vi "Intensity_png.vi"(3 "No of Contours":i32=20, 4 "Job Directory":path=path "/Lacie_20/paulhayden/Documents/EnFlo bits/EnFlo Tun Vel profiles/View_LDA data.tpt", 5 "Intensity Graph":dbl[][](graph)) -> ()   [LabVIEW 2018]
uses:
  Results_plotter_Global.vi
panel:
  out "Folders":string[](array[string])
  out "String":string
  in  "Added labels":i32[](listbox)
  in  "Z Min":dbl=0.97
  in  "Z Max":dbl=1.07
  in  "Save Automatically?":bool
  in  "Auto scale Intensity":bool=TRUE
  in  "Colour":bool=TRUE
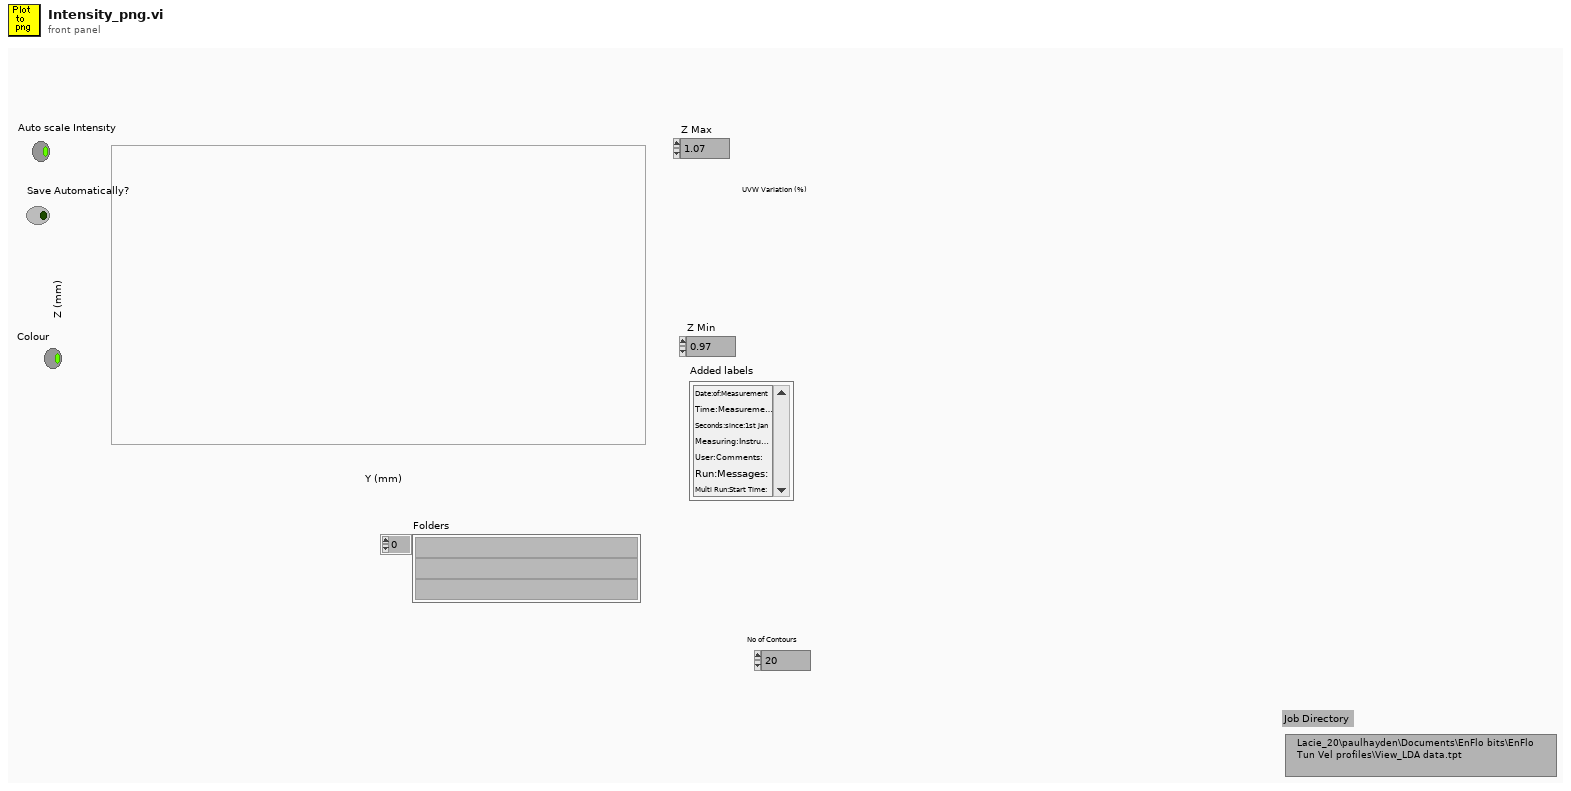
[diagram p1: front panel]
types:
  T1 = typedef "imagedata.ctl" = cluster{"image type":i32, "image depth":i32, "image":u8[], "mask":u8[], "colors":u32[], "Rectangle":cluster{"left":i16, "top":i16, "right":i16, "bottom":i16}}
  T2 = cluster{"left":i16, "top":i16, "right":i16, "bottom":i16}
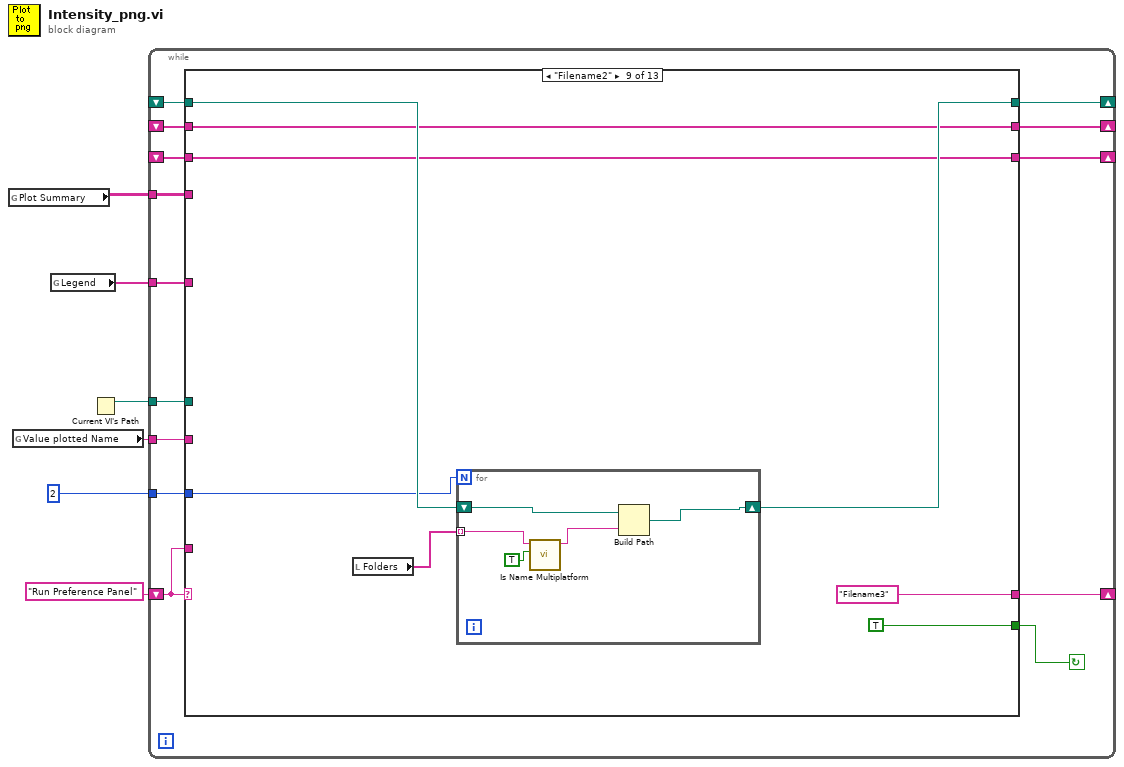
[diagram p0: block diagram]
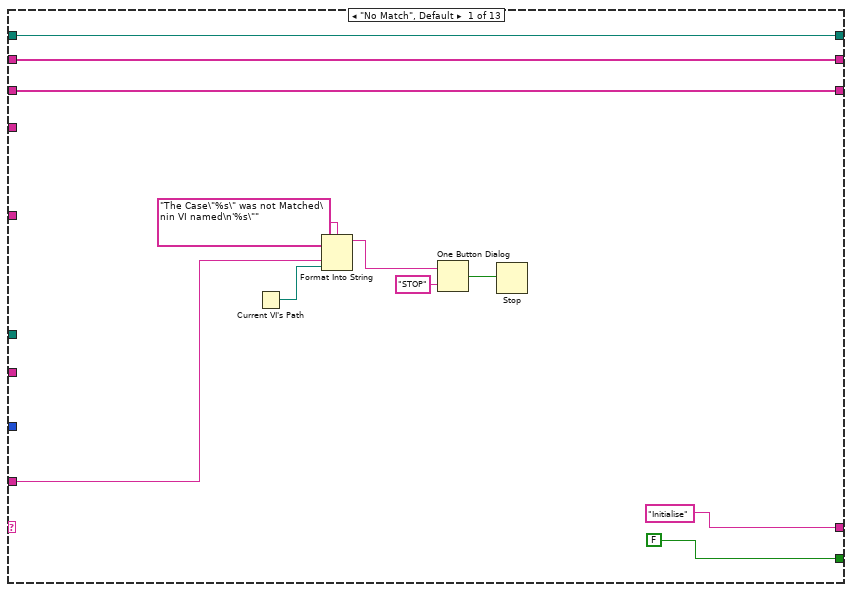
[diagram p2: hidden frame]
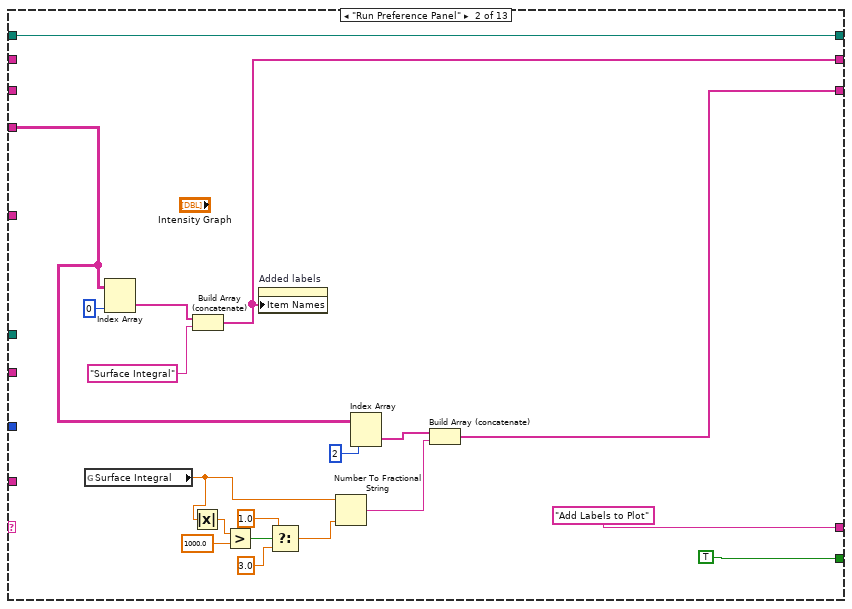
[diagram p3: hidden frame]
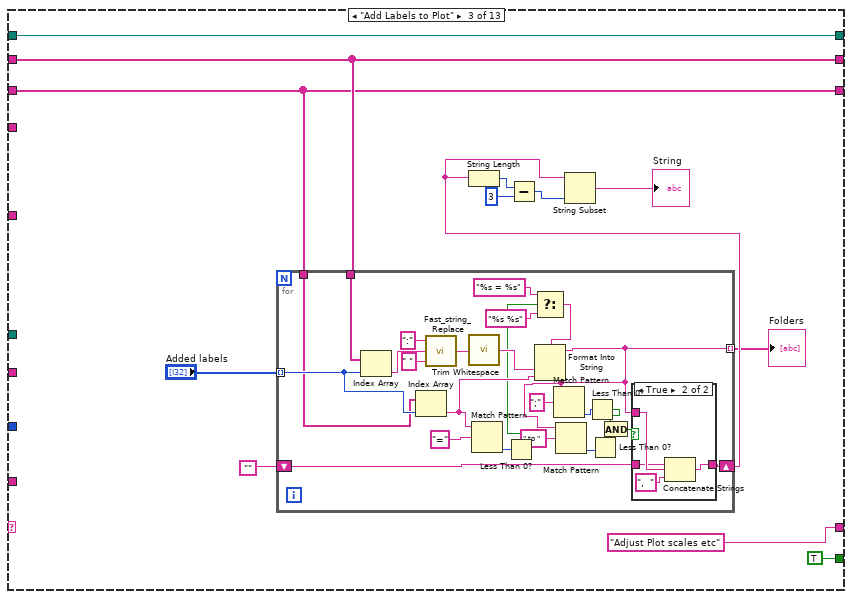
[diagram p4: hidden frame]
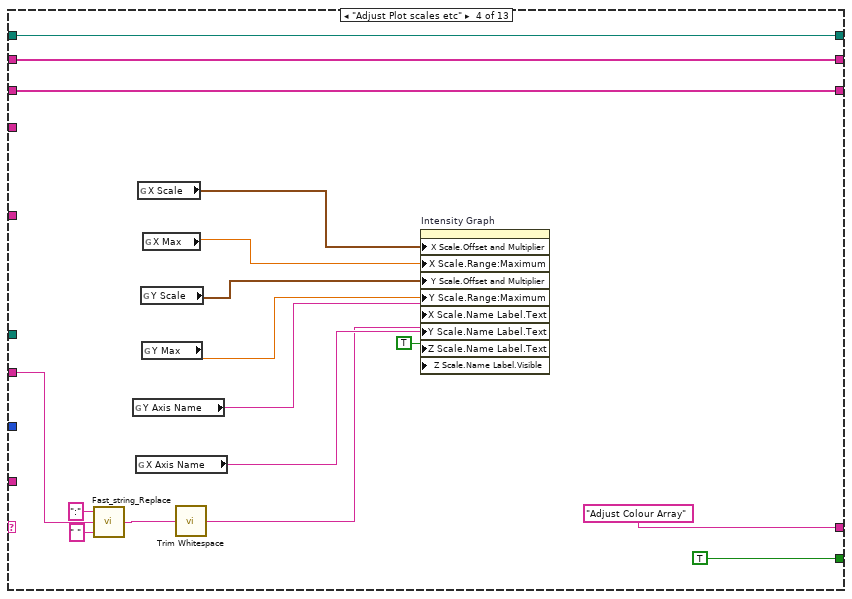
[diagram p6: hidden frame]
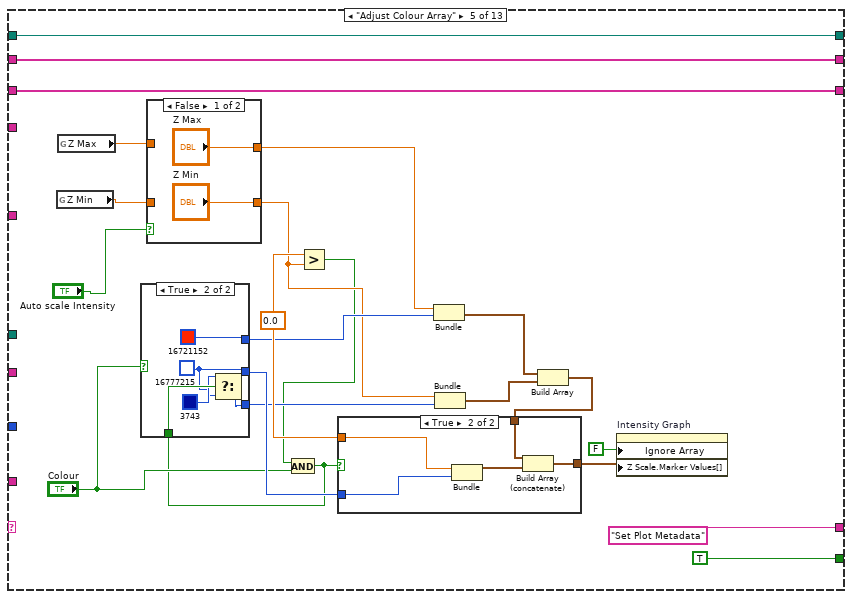
[diagram p7: hidden frame]
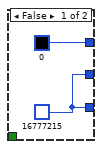
[diagram p8: hidden frame]
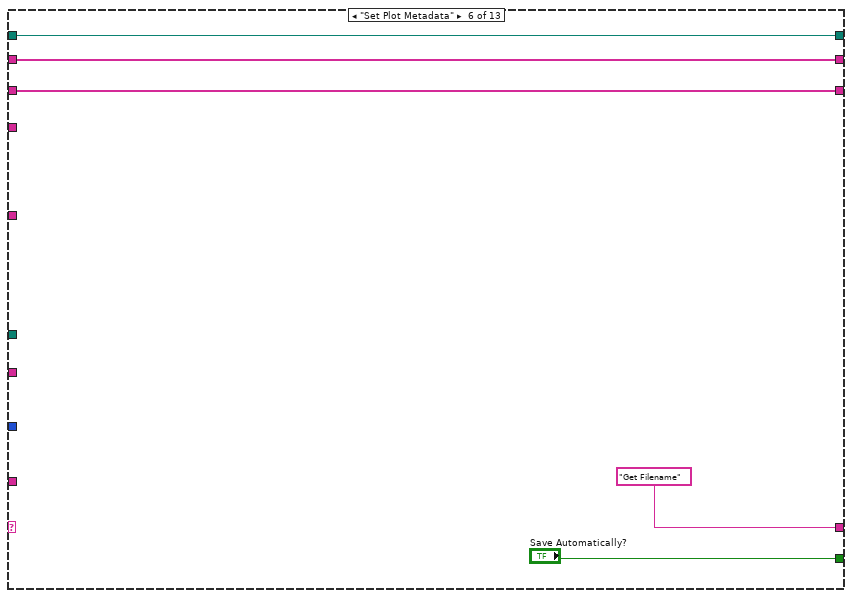
[diagram p11: hidden frame]
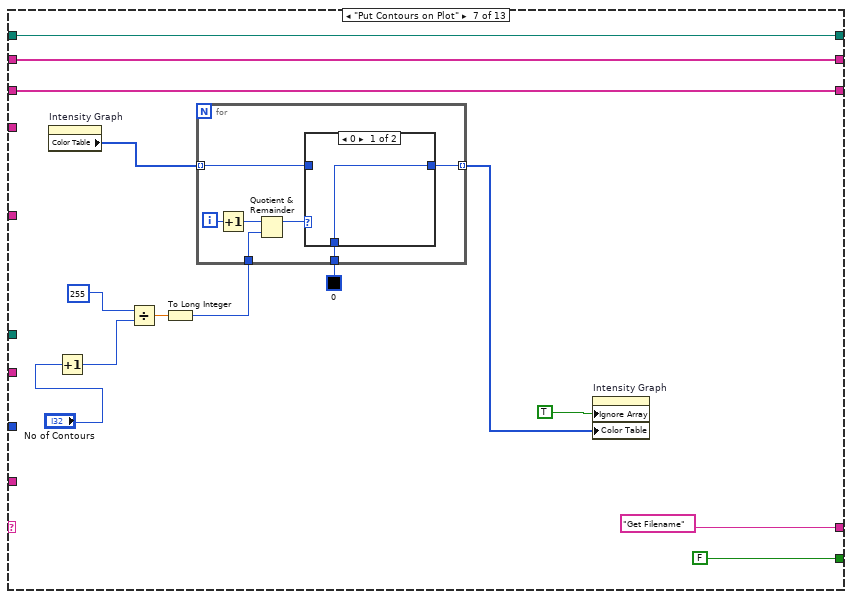
[diagram p12: hidden frame]
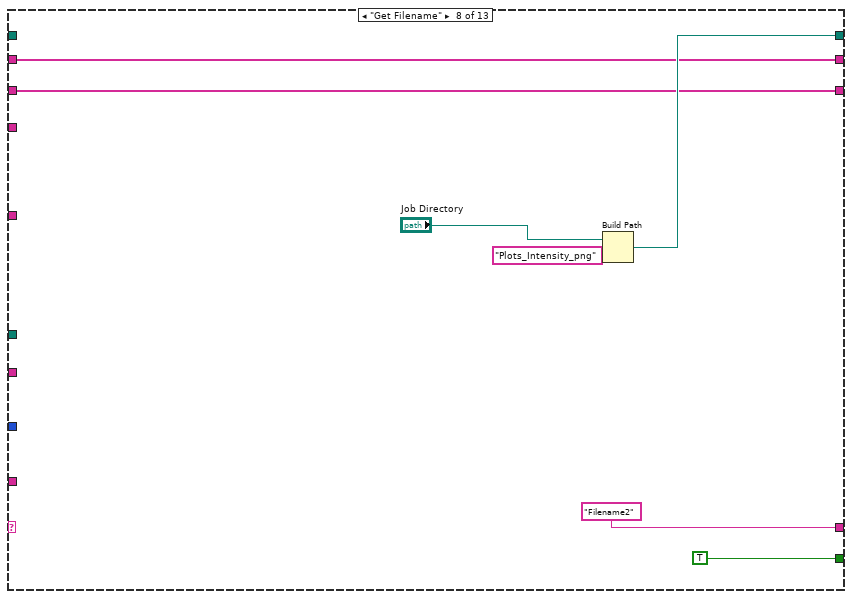
[diagram p14: hidden frame]
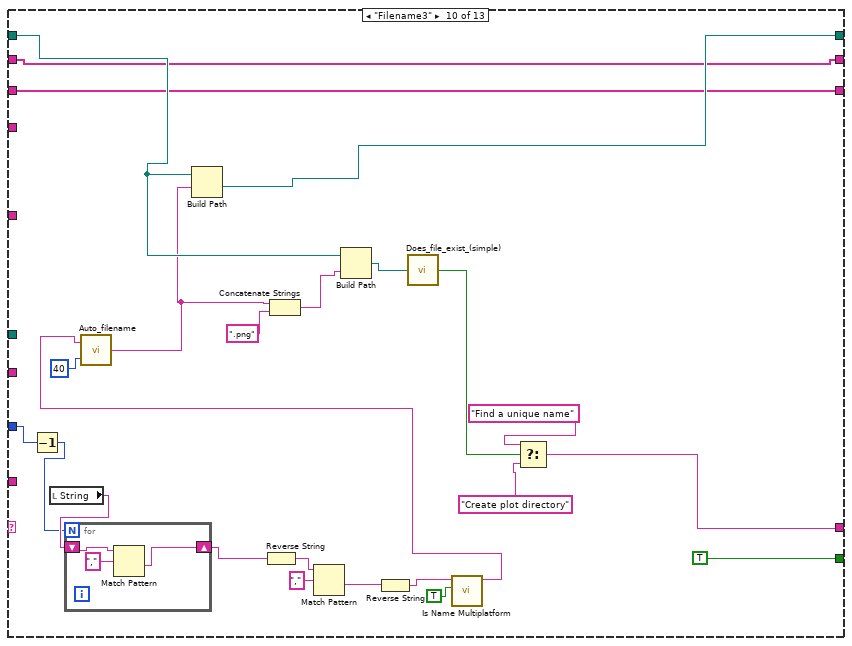
[diagram p15: hidden frame]
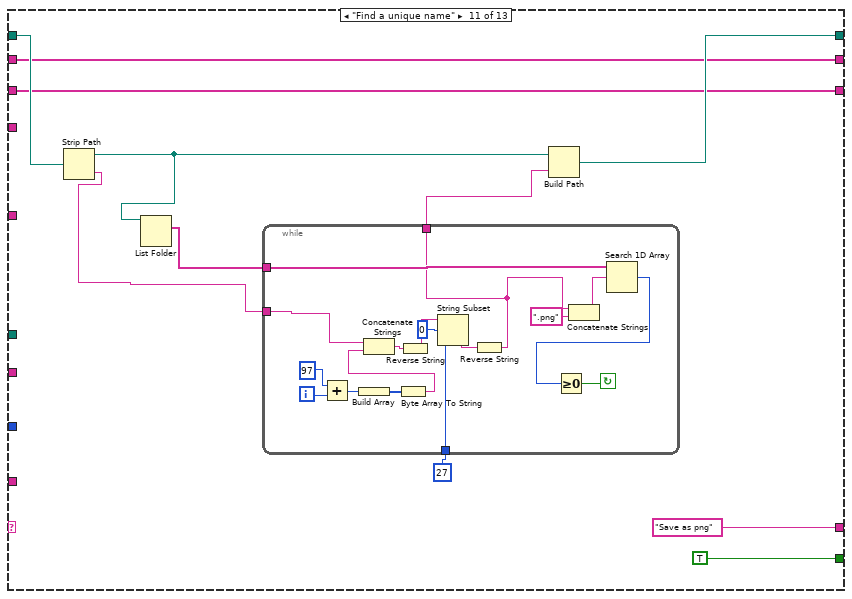
[diagram p16: hidden frame]
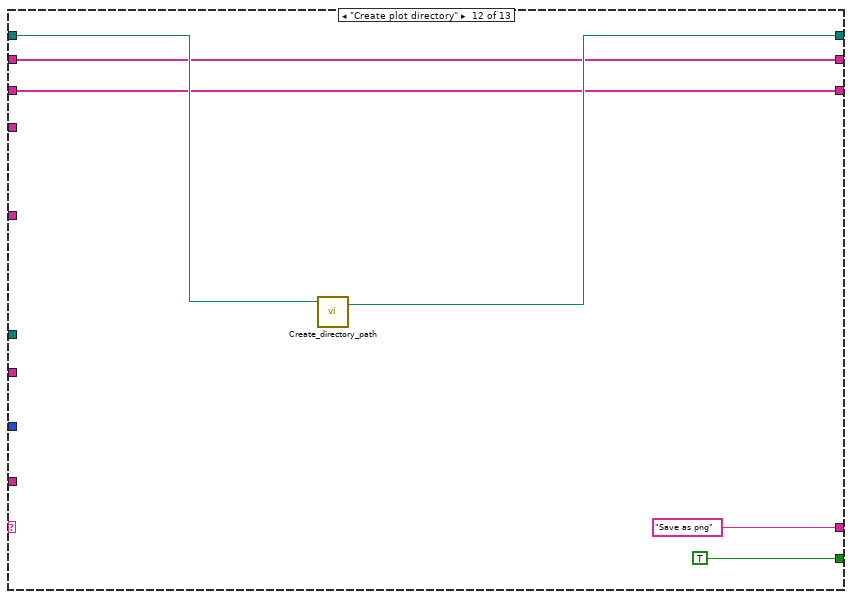
[diagram p17: hidden frame]
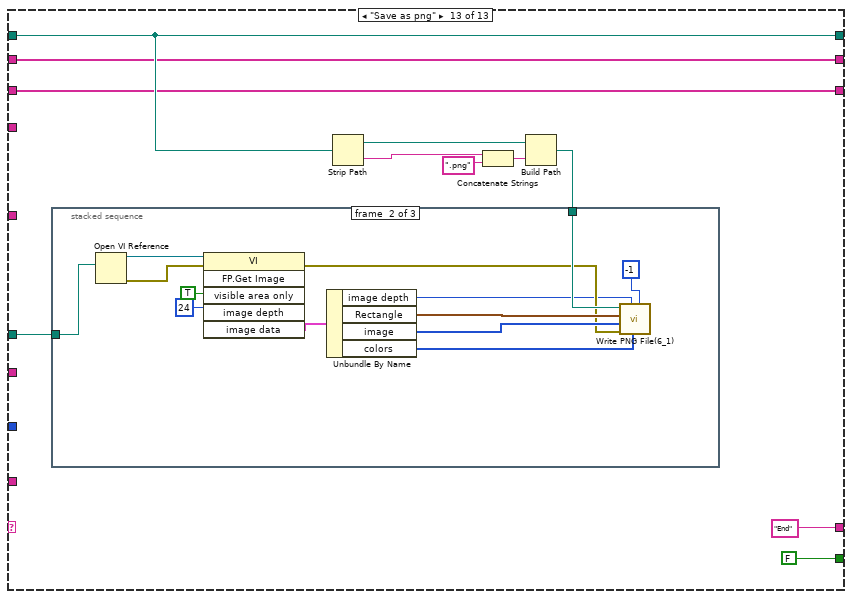
[diagram p18: hidden frame]
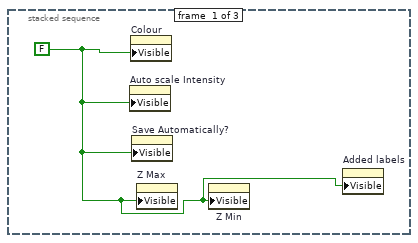
[diagram p19: hidden frame]
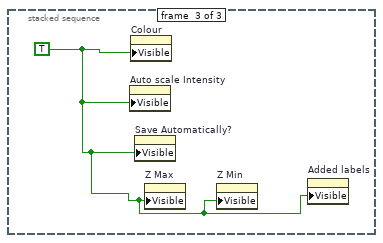
[diagram p20: hidden frame]
diagram:
  n1 = global read "Results_plotter_Global.vi" "Plot Summary"() -> (w2:string[][])
  n2 = global read "Results_plotter_Global.vi" "Value plotted Name"() -> (w4:string)
  n3 = global read "Results_plotter_Global.vi" "Legend"() -> (w3:string[])
  n4 = Current VI's Path() -> (path=w5:path)
  n5 = while {
    shift-left: "Run Preference Panel" -> [w18]
    shift-right: [w19] -> _
    tunnel: w5 -> [w17]
    shift-right: [w16] -> _
    shift-left: _ -> [w15]
    tunnel: w4 -> [w14]
    tunnel: w3 -> [w13]
    tunnel: w2 -> [w12]
    tunnel: 2 -> [w11]
    shift-right: [w10] -> _
    shift-left: _ -> [w8]
    shift-right: [w9] -> _
    shift-left: _ -> [w7]
    stop <- w20 continue-if-true
    n6 = case shown="\"Filename2\"" w18 {
      tunnel: [FALSE TRUE TRUE ("Top Level") TRUE ("Top Level") TRUE ("Top Level") "Save Automatically?" FALSE ("Top Level") TRUE ("Top Level") TRUE ("Top Level") TRUE ("Top Level") TRUE ("Top Level") TRUE ("Top Level") FALSE ("Top Level")] -> w20
      tunnel: ["Initialise" "Add Labels to Plot" "Adjust Plot scales etc" "Adjust Colour Array" "Set Plot Metadata" "Get Filename" "Get Filename" "Filename2" "Filename3" w218 "Save as png" "Save as png" "End"] -> w19
      tunnel: w18 -> [w26 _ _ _ _ _ _ _ _ _ _ _ _]
      tunnel: w17 -> [_ _ _ _ _ _ _ _ _ _ _ _ w268]
      tunnel: [w23 w48 w62 w101 w121 w153 w157 w182 w188 w219 w229 w255 w266] -> w16
      tunnel: w15 -> [w23 w48 w62 w101 w121 w153 w157 _ w190 w220 w230 w256 w266]
      tunnel: w14 -> [_ _ _ w100 _ _ _ _ _ _ _ _ _]
      tunnel: w13 -> [_ _ _ _ _ _ _ _ _ _ _ _ _]
      tunnel: w12 -> [_ w42 _ _ _ _ _ _ _ _ _ _ _]
      tunnel: w11 -> [_ _ _ _ _ _ _ _ w187 w204 _ _ _]
      tunnel: [w22 w44 w52 w95 w112 w151 w156 w179 w186 w202 w226 w254 w262] -> w10
      tunnel: [w21 w39 w51 w94 w111 w150 w155 w178 w185 w201 w225 w253 w261] -> w9
      tunnel: w8 -> [w22 _ w52 w95 w112 w151 w156 w179 w186 w202 w226 w254 w262]
      tunnel: w7 -> [w21 _ w51 w94 w111 w150 w155 w178 w185 w201 w225 w253 w261]
      frame "No Match", Default {
        n7 = Current VI's Path() -> (path=w25:path)
        n8 = Format Into String(format string="The Case\"%s\" was not Matched\nin VI named\n'%s\"" ("Format String"), w26, w25) -> (resulting string=w29:string)  [unwired: 2 in, 1 out]
        n9 = One Button Dialog(message=w29, button name ("OK")="STOP") -> (true=w27:bool)
        n10 = Stop(stop? (T)=w27) -> ()
      }
      frame "Run Preference Panel" {
        n11 = global read "Results_plotter_Global.vi" "Surface Integral"() -> (w33:dbl)
        n12 = Index Array(array=w42, index (col)=0 ("disabled index (col)")) -> (element=w46:string[])  [unwired: 1 in]
        n13 = Absolute Value(x=w33) -> (abs(x)=w32:dbl)
        n14 = Build Array (concatenate)(w46, "Surface Integral" ("Output String")) -> (w44:string[])
        n15 = Greater?(x=w32, y=1000.0) -> (0:w37:bool)
        n16 = property on="Added labels" class="LstBox (strict)"("Item Names"=w44) -> ()  [unwired: 2 in, 2 out]
        n17 = Select(t=1.0, s=w37, f=3.0) -> (s? t:f=w36:dbl)
        n18 = Number To Fractional String(number=w33, precision (6)=w36) -> (F-format string=w41:string)  [unwired: 2 in]
        n19 = Index Array(array=w42, index (col)=2 ("disabled index (col)")) -> (element=w40:string[])  [unwired: 1 in]
        n20 = Build Array (concatenate)(w40, w41) -> (w39:string[])
      }
      frame "Add Labels to Plot" {
        n21 = for {
          tunnel: "Added labels" -> [w87] mode=indexing
          tunnel: w52 -> [w88]
          shift-right: [w79] -> w55
          shift-left: "" -> [w80]
          tunnel: [w65] -> w53 mode=indexing
          tunnel: w51 -> [w64]
          n22 = Index Array(array=w88, index=w87) -> (element=w84:string)
          n23 = Index Array(array=w64, index=w87) -> (element=w78:string)
          n24 = call "Fast_string_Replace.vi"("Replace match with:"=" ", "Input String"=w84, "regular expression"=":") -> ("Output String"=w83:string)  [unwired: 2 out]
          n25 = call <vilib>:"Trim Whitespace.vi"("string"=w83) -> ("trimmed string"=w82:string)  [unwired: 1 in]
          n26 = Match Pattern(string=w78, regular expression="=") -> (offset past match=w76:i32)  [unwired: 4 out]
          n27 = Less Than 0?(x=w76) -> (x < 0?=w75:bool)
          n28 = Select(t="%s = %s" ("format string"), s=w75, f="%s %s" ("format string")) -> (s? t:f=w72:string)
          n29 = Format Into String(format string=w72, w82, w78) -> (resulting string=w65:string)  [unwired: 2 in, 1 out]
          n30 = Match Pattern(string=w65, regular expression=";") -> (offset past match=w70:i32)  [unwired: 4 out]
          n31 = Match Pattern(string=w65, regular expression=" to ") -> (offset past match=w69:i32)  [unwired: 4 out]
          n32 = Less Than 0?(x=w70) -> (x < 0?=w67:bool)
          n33 = Less Than 0?(x=w69) -> (x < 0?=w68:bool)
          n34 = And(x=w67, y=w68) -> (x .and. y?=w66:bool)
          n35 = case shown="True" w66 {
            tunnel: w80 -> [w89 w91]
            tunnel: [w89 w92] -> w79
            tunnel: w65 -> [_ w93]
            frame False {
            }
            frame True {
              n36 = Concatenate Strings(w91, w93, ",  " ("string")) -> (w92:string)
            }
          }
        }
        "Folders" <- w53
        n37 = String Length(string=w55) -> (length=w58:i32)
        n38 = Subtract(x=w58, y=3) -> (x-y=w56:i32)
        n39 = String Subset(string=w55, length (rest)=w56) -> (substring=→"String":string)  [unwired: 1 in]
      }
      frame "Adjust Plot scales etc" {
        n40 = call "Fast_string_Replace.vi"("Replace match with:"=" ", "Input String"=w100, "regular expression"=":") -> ("Output String"=w97:string)  [unwired: 1 in, 1 out]
        n41 = global read "Results_plotter_Global.vi" "Y Axis Name"() -> (w104:string)
        n42 = global read "Results_plotter_Global.vi" "X Axis Name"() -> (w103:string)
        n43 = global read "Results_plotter_Global.vi" "X Scale"() -> (w109:cluster{"Xo":dbl, "delta X":dbl})
        n44 = global read "Results_plotter_Global.vi" "Y Scale"() -> (w107:cluster{"Xo":dbl, "delta X":dbl})
        n45 = global read "Results_plotter_Global.vi" "Y Max"() -> (w106:dbl)
        n46 = global read "Results_plotter_Global.vi" "X Max"() -> (w108:dbl)
        n47 = call <vilib>:"Trim Whitespace.vi"("string"=w97) -> ("trimmed string"=w96:string)  [unwired: 1 in]
        n48 = property on="Intensity Graph" class="IntGraph (strict)"("X Scale.Offset and Multiplier"=w109, "X Scale.Range:Maximum"=w108, "Y Scale.Offset and Multiplier"=w107, "Y Scale.Range:Maximum"=w106, "X Scale.Name Label.Text"=w104, "Y Scale.Name Label.Text"=w103, "Z Scale.Name Label.Text"=w96, "Z Scale.Name Label.Visible"=TRUE) -> ()  [unwired: 2 in, 2 out]
      }
      frame "Adjust Colour Array" {
        w132 = 0.0 ("max Z value")
        n49 = global read "Results_plotter_Global.vi" "Z Min"() -> (w117:dbl)
        n50 = global read "Results_plotter_Global.vi" "Z Max"() -> (w119:dbl)
        n51 = case shown="False" "Auto scale Intensity" {
          tunnel: ["Z Max" w143] -> w120
          tunnel: w119 -> [_ w143]
          tunnel: ["Z Min" w142] -> w118
          tunnel: w117 -> [_ w142]
          frame False {
          }
          frame True {
          }
        }
        n52 = Greater?(x=w132, y=w118) -> (0:w115:bool)
        n53 = And(x=w115, y="Colour") -> (x .and. y?=w113:bool)
        n54 = case shown="True" "Colour" {
          tunnel: [w134 w135] -> w128
          tunnel: [u32 0 u32 16721152] -> w127
          tunnel: [w134 w136] -> w123
          tunnel: w113 -> [_ w138]
          frame False {
            w134 = u32 16777215
          }
          frame True {
            w135 = u32 16777215
            n55 = Select(t=u32 3743, s=w138, f=w135) -> (s? t:f=w136:u32)
          }
        }
        n56 = Bundle("Z Max"=w120, w127) -> (w129:cluster{"Z Max":dbl, u32})  [unwired: 1 in]
        n57 = Bundle("Z Min"=w118, w123) -> (w131:cluster{"Z Min":dbl, u32})  [unwired: 1 in]
        n58 = Build Array(w129, w131) -> (w130:cluster{"Z Min":dbl, u32}[])
        n59 = case shown="True" w113 {
          tunnel: w130 -> [w144 w149]
          tunnel: [w144 w147] -> w125
          tunnel: w128 -> [_ w146]
          tunnel: w132 -> [_ w145]
          frame False {
          }
          frame True {
            n60 = Bundle("max Z value"=w145, w146) -> (w148:cluster{"max Z value":dbl, u32})  [unwired: 1 in]
            n61 = Build Array (concatenate)(w149, w148) -> (w147:cluster{"max Z value":dbl, u32}[])
          }
        }
        n62 = property on="Intensity Graph" class="IntGraph (strict)"("Ignore Array"=FALSE, "Z Scale.Marker Values[]"=w125) -> ()  [unwired: 2 in, 2 out]
      }
      frame "Set Plot Metadata" {
      }
      frame "Put Contours on Plot" {
        n63 = property on="Intensity Graph" class="IntGraph (strict)"() -> ("Color Table"=w160:u32[])  [unwired: 2 in, 2 out]
        n64 = Increment(x="No of Contours") -> (x+1=w165:i32)
        n65 = Divide(x=255, y=w165) -> (x/y=w164:dbl)
        n66 = To Long Integer(number=w164) -> (32bit integer=w162:i32)
        n67 = for {
          tunnel: w162 -> [w174]
          tunnel: [w171] -> w159 mode=indexing
          tunnel: w160 -> [w170] mode=indexing
          tunnel: u32 0 -> [w169]
          i -> [w175]
          n68 = Increment(x=w175) -> (x+1=w172:i32)
          n69 = Quotient & Remainder(x=w172, y=w174) -> (x-y*floor(x/y)=w173:i32)  [unwired: 1 out]
          n70 = case shown="0" w173 {
            tunnel: [w176 w177] -> w171
            tunnel: w170 -> [_ w177]
            tunnel: w169 -> [w176 _]
            frame 0 {
            }
            frame 1, Default {
            }
          }
        }
        n71 = property on="Intensity Graph" class="IntGraph (strict)"("Ignore Array"=TRUE, "Color Table"=w159) -> ()  [unwired: 2 in, 2 out]
      }
      frame "Get Filename" {
        n72 = Build Path(base path="Job Directory", name or relative path="Plots_Intensity_png") -> (appended path=w182:path)
      }
      frame "Filename2" {
        n73 = local read "Folders"() -> (w189:string[])
        n74 = for {
          N: w187 -> [_]
          shift-right: [w196] -> w188
          shift-left: w190 -> [w197]
          tunnel: w189 -> [w194] mode=indexing
          n75 = call <vilib>:"Is Name Multiplatform.vi"("filename must be valid on all platforms (F)"=TRUE ("name must work for all platforms (F)"), "filename"=w194) -> ("suggested filename"=w193:string)  [unwired: 5 in, 4 out]
          n76 = Build Path(base path=w197, name or relative path=w193) -> (appended path=w196:path)
        }
      }
      frame "Filename3" {
        n77 = Decrement(x=w204) -> (x-1=w203:i32)
        n78 = local read "String"() -> (w206:string)
        n79 = for {
          N: w203 -> [_]
          shift-right: [w222] -> w205
          shift-left: w206 -> [w223]
          n80 = Match Pattern(string=w223, regular expression=",") -> (after substring=w222:string)  [unwired: 1 in, 3 out]
        }
        n81 = Reverse String(1:w205) -> (0:w208:string)
        n82 = Match Pattern(string=w208, regular expression=",") -> (after substring=w207:string)  [unwired: 1 in, 3 out]
        n83 = Reverse String(1:w207) -> (0:w199:string)
        n84 = call <vilib>:"Is Name Multiplatform.vi"("filename must be valid on all platforms (F)"=TRUE ("name must work for all platforms (F)"), "filename"=w199) -> ("suggested filename"=w198:string)  [unwired: 5 in, 4 out]
        n85 = call "Auto_filename.vi"("Filename Max length"=40, "Prefix"=w198) -> ("Filename"=w211:string)
        n86 = Build Path(base path=w220, name or relative path=w211) -> (appended path=w219:path)
        n87 = Concatenate Strings(w211, ".png" ("string")) -> (w216:string)
        n88 = Build Path(base path=w220, name or relative path=w216) -> (appended path=w215:path)
        n89 = call "Does_file_exist_(simple).vi"("Pathname"=w215) -> ("exists?"=w214:bool)
        n90 = Select(t="Find a unique name", s=w214, f="Create plot directory") -> (s? t:f=w218:string)
      }
      frame "Find a unique name" {
        n91 = Strip Path(path=w230) -> (stripped path=w228:path, name=w232:string)
        n92 = List Folder(path=w228) -> (filenames=w227:string[])  [unwired: 3 in, 3 out]
        n93 = while {
          tunnel: w232 -> [w252]
          tunnel: 27 ("Max Length") -> [w251]
          tunnel: [w237] -> w233
          tunnel: w227 -> [w241]
          i -> [w242]
          stop <- w239 continue-if-true
          n94 = Add(x=97, y=w242) -> (x+y=w249:i32)
          n95 = Build Array(w249) -> (w250:i32[])
          n96 = Byte Array To String(unsigned byte array=w250) -> (string=w247:string)
          n97 = Concatenate Strings(w252, w247) -> (w245:string)
          n98 = Reverse String(1:w245) -> (0:w246:string)
          n99 = String Subset(string=w246, offset (0)=0, length (rest)=w251) -> (substring=w244:string)
          n100 = Reverse String(1:w244) -> (0:w237:string)
          n101 = Concatenate Strings(w237, ".png" ("string")) -> (w236:string)
          n102 = Search 1D Array(1D array=w241, element=w236) -> (index of element=w240:i32)  [unwired: 1 in]
          n103 = Greater Or Equal To 0?(x=w240) -> (x >= 0?=w239:bool)
        }
        n104 = Build Path(base path=w228, name or relative path=w233) -> (appended path=w229:path)
      }
      frame "Create plot directory" {
        n105 = call "Create_directory_path.vi"("Path name"=w256) -> ("Path name Out"=w255:path)  [unwired: 2 in, 1 out]
      }
      frame "Save as png" {
        n106 = Strip Path(path=w266) -> (stripped path=w259:path, name=w260:string)
        n107 = Concatenate Strings(w260, ".png" ("string")) -> (w265:string)
        n108 = Build Path(base path=w259, name or relative path=w265) -> (appended path=w263:path)
        n109 = stacked-sequence {
          tunnel: w268 -> [_ w281 _]
          tunnel: w263 -> [_ w279 _]
          frame #0 {
            w270 = FALSE ("Visible")
            n110 = property on="Auto scale Intensity" class="Bool (strict)"("Visible"=w270) -> ()  [unwired: 2 in, 2 out]
            n111 = property on="Colour" class="Bool (strict)"("Visible"=w270) -> ()  [unwired: 2 in, 2 out]
            n112 = property on="Save Automatically?" class="Bool (strict)"("Visible"=w270) -> ()  [unwired: 2 in, 2 out]
            n113 = property on="Z Max" class="DigNum (strict)"("Visible"=w270) -> ()  [unwired: 2 in, 2 out]
            n114 = property on="Z Min" class="DigNum (strict)"("Visible"=w270) -> ()  [unwired: 2 in, 2 out]
            n115 = property on="Added labels" class="LstBox (strict)"("Visible"=w270) -> ()  [unwired: 2 in, 2 out]
          }
          frame #1 {
            n116 = Open VI Reference(vi path=w281) -> (vi reference=w283:refnum<vi>, error out=w282:errorcluster)  [unwired: 5 in]
            n117 = invoke class="VI" method="FP.Get Image"(reference=w283, error in=w282, "visible area only"=TRUE, "image depth"=24 ("Image Depth")) -> (error out=w274:errorcluster, "image data"=w272:T1)  [unwired: 2 in, 4 out]
            n118 = Unbundle By Name(w272) -> ("image depth"=w273:i32, "Rectangle"=w277:T2, "image"=w278:u8[], "colors"=w275:u32[])
            n119 = call <vilib>:"Write PNG File(6_1).vi"("compression (default)"=-1, "color table"=w275, "depth"=w273, "error in (no error)"=w274, "flattened image data"=w278, "rect"=w277, "path to PNG file"=w279) -> ()  [unwired: 3 in, 2 out]
          }
          frame #2 {
            w284 = TRUE ("Visible")
            n120 = property on="Auto scale Intensity" class="Bool (strict)"("Visible"=w284) -> ()  [unwired: 2 in, 2 out]
            n121 = property on="Colour" class="Bool (strict)"("Visible"=w284) -> ()  [unwired: 2 in, 2 out]
            n122 = property on="Save Automatically?" class="Bool (strict)"("Visible"=w284) -> ()  [unwired: 2 in, 2 out]
            n123 = property on="Z Max" class="DigNum (strict)"("Visible"=w284) -> ()  [unwired: 2 in, 2 out]
            n124 = property on="Z Min" class="DigNum (strict)"("Visible"=w284) -> ()  [unwired: 2 in, 2 out]
            n125 = property on="Added labels" class="LstBox (strict)"("Visible"=w284) -> ()  [unwired: 2 in, 2 out]
          }
        }
      }
    }
  }
